vi "infer.vi"() -> ()   [LabVIEW 2013]
panel:
  in  "Movement data from both players 2":i32[][](array[numeric])
  in  "end 2":i32[](array[numeric])
  in  "start 2":i32[](array[numeric])
  out "Infered action indicators":string[][](array[string])
  out "Numeric":i32
  out "Array":string[][](array[string])
  in  "end":i32[](array[numeric])=[898, 1265, 1783, 2060, 2244, 2535, 2836, 2998, 3152, 3333, 3625, 3861, 4157, 4419, 4737, 4931, 5183, 5355, 5532, 5686, 5939, 6561, 6729, 6902, 7174, 7421, 7716, 7925, 8223, 8442, 8667, 8996, 9247, 9451, 9730, 9993, 10191, 10366, 10617]
  in  "start":i32[](array[numeric])=[845, 1034, 1720, 1941, 2200, 2401, 2787, 2982, 3135, 3271, 3450, 3828, 4017, 4351, 4642, 4893, 5127, 5332, 5484, 5654, 5831, 6518, 6681, 6854, 7105, 7330, 7627, 7891, 8116, 8404, 8588, 8839, 9180, 9394, 9661, 9952, 10139, 10317, 10523]
  in  "Movement data from both players":i32[][](array[numeric])=array10719x2[21438 elements]
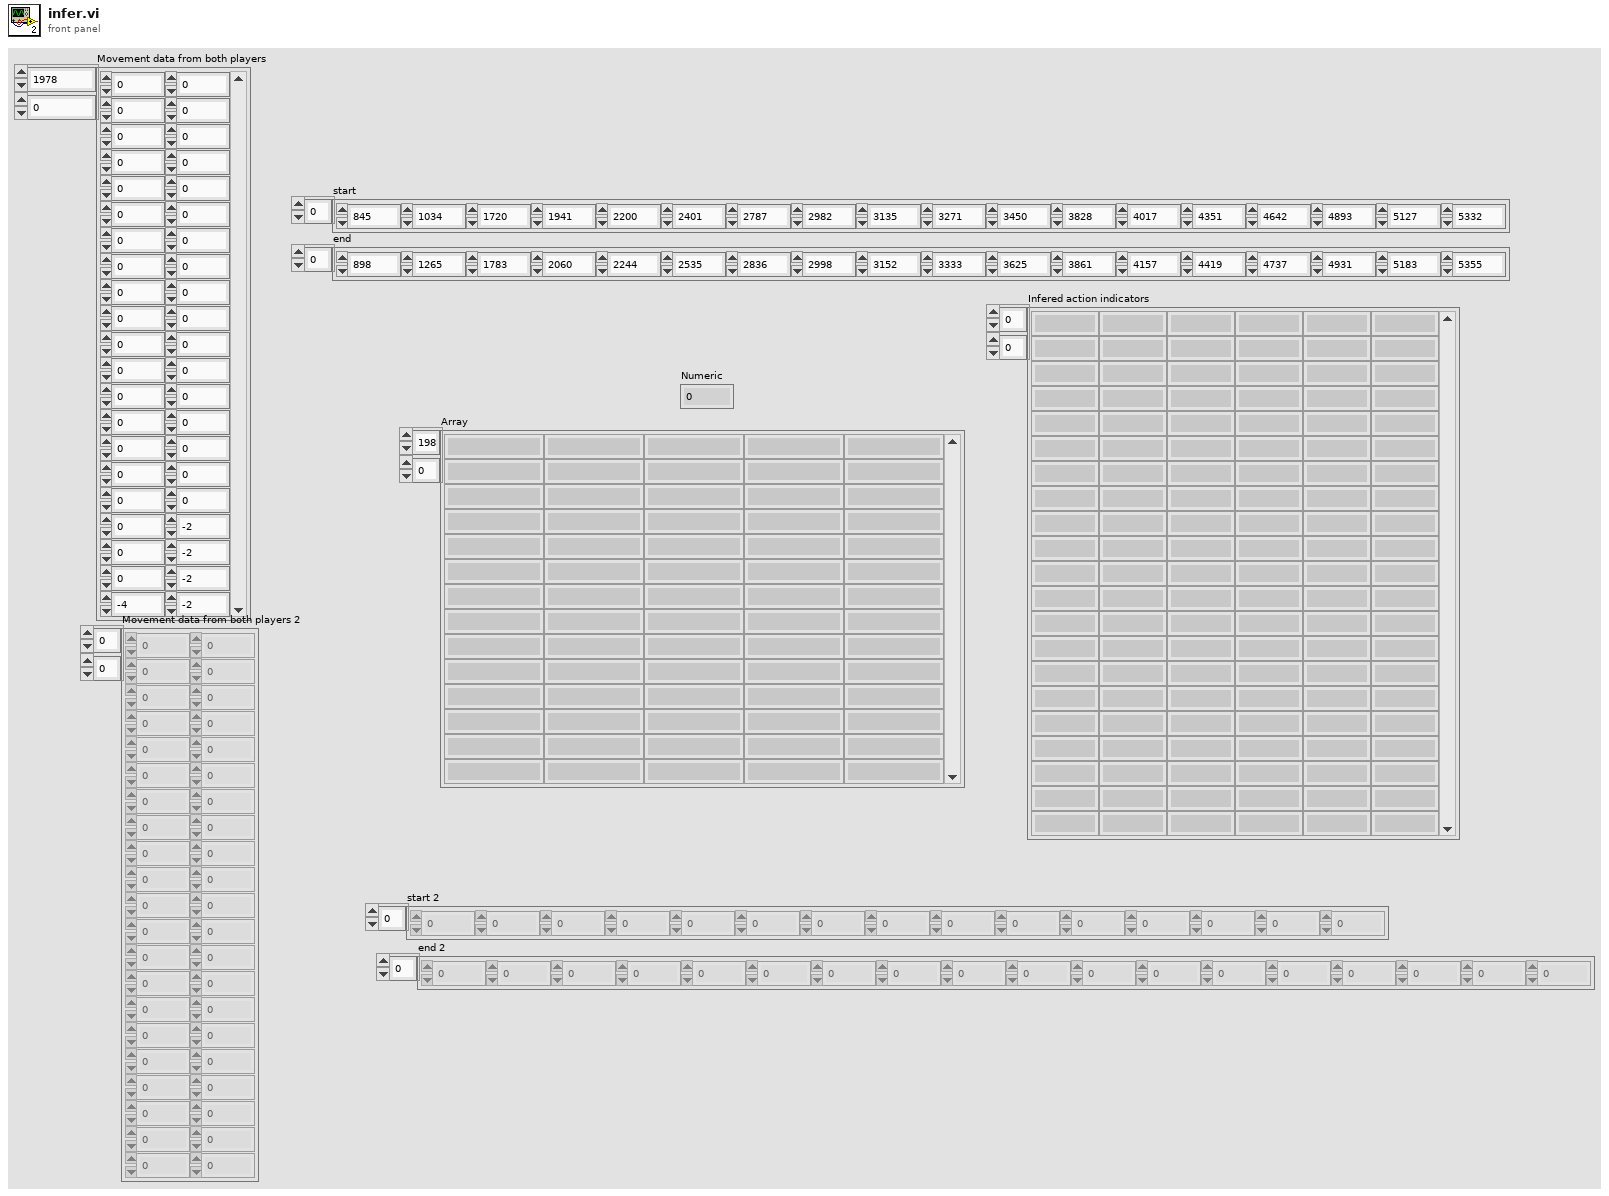
[diagram p1: front panel]
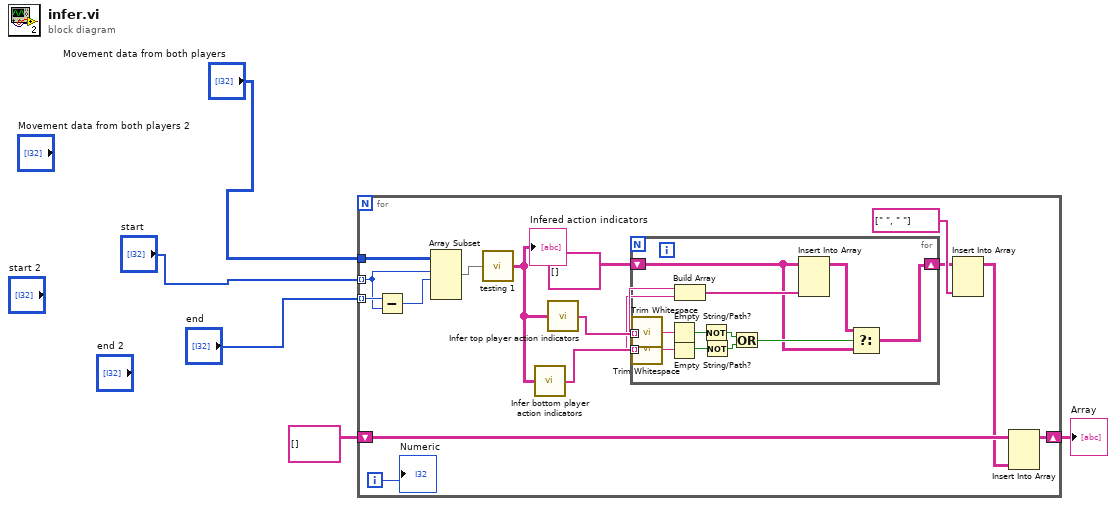
[diagram p0: block diagram]
diagram:
  n1 = for {
    tunnel: "start" -> [w19] mode=indexing
    tunnel: "end" -> [w20] mode=indexing
    tunnel: "Movement data from both players" -> [w10]
    shift-right: [w13] -> w4
    shift-left: string[][] [] -> [w14]
    i -> [w11]
    n2 = Subtract(x=w20, y=w19) -> (x-y=w18:i32)
    n3 = Array Subset(array=w10, index (row)=w19, length (row)=w18) -> (w7:i32[][])  [unwired: 2 in]
    n4 = call "testing 1.vi"("movement data from both players"=w7) -> ("Infered action indicators"=w9:string[][])
    "Infered action indicators" <- w9
    n5 = call "Infer bottom player action indicators.vi"("Movement data with player transitions notated"=w9) -> ("Bottom player infered actions column"=w8:string[])
    n6 = call "Infer top player action indicators.vi"("Movement data with player transitions notated"=w9) -> ("Top player infered actions column"=w6:string[])
    n7 = for {
      tunnel: w6 -> [w26] mode=indexing
      tunnel: w8 -> [w25] mode=indexing
      shift-right: [w21] -> w16
      shift-left: string[][] [] -> [w22]
      n8 = call <vilib>:"Trim Whitespace.vi"("string"=w26) -> ("trimmed string"=w33:string)  [unwired: 1 in]
      n9 = call <vilib>:"Trim Whitespace.vi"("string"=w25) -> ("trimmed string"=w32:string)  [unwired: 1 in]
      n10 = Empty String/Path?(string/path=w33) -> (empty?=w31:bool)
      n11 = Empty String/Path?(string/path=w32) -> (empty?=w30:bool)
      n12 = Build Array(w26, w25) -> (w24:string[])
      n13 = Not(x=w31) -> (.not. x?=w28:bool)
      n14 = Not(x=w30) -> (.not. x?=w29:bool)
      n15 = Or(x=w28, y=w29) -> (x .or. y?=w27:bool)
      n16 = Insert Into Array(array=w22, new element=w24) -> (w23:string[][])  [unwired: 2 in]
      n17 = Select(t=w23, s=w27, f=w22) -> (s? t:f=w21:string[][])
    }
    n18 = Insert Into Array(array=w16, new element=string[] [" ", " "] ("new element/subarray")) -> (w12:string[][])  [unwired: 2 in]
    n19 = Insert Into Array(array=w14, new element=w12) -> (w13:string[][])  [unwired: 2 in]
    "Numeric" <- w11
  }
  "Array" <- w4
